vi "DriveModuleControl_TravTunePID-ALT.vi"(8 "error in":errorcluster, 9 "Actual State":T1={"Speed"=0.0, "Angle"={"VALUE"=0.0, "COS"=1.0, "SIN"=0.0}} {"Angle"."SIN" format="%13.4f"; "Angle"."COS" format="%13.4f"; "Angle"."VALUE" format="%13.4f"}, 10 "Desired State":T1={"Speed"=0.0, "Angle"={"VALUE"=0.0, "COS"=1.0, "SIN"=0.0}} {"Angle"."SIN" format="%13.4f"; "Angle"."COS" format="%13.4f"; "Angle"."VALUE" format="%13.4f"}, 11 "ModualNamePrefix":i32) -> (0 "error out":errorcluster)   [LabVIEW 2023]
uses:
  <vilib>/Rock Robotics/WPI/ThirdParty/JAS_Junk/TrajLib/TypeDef/SWERVE_DRIVE_MODULE_STATE.ctl
  <vilib>/Rock Robotics/WPI/ThirdParty/JAS_Junk/TrajLib/TypeDef/ROTATION2D.ctl
  <vilib>/Rock Robotics/WPI/ThirdParty/JAS_Junk/TrajLib/Rotation2d_Minus.vi
  <vilib>/Rock Robotics/WPI/ThirdParty/JAS_Junk/TrajLib/Rotation2d_GetRadians.vi
  <vilib>/Rock Robotics/WPI/ThirdParty/JAS_Junk/TrajLib/SwerveModuleState_New.vi
  <vilib>/Rock Robotics/WPI/ThirdParty/JAS_Junk/TrajLib/Rotation2d_RotateBy.vi
  <vilib>/Rock Robotics/WPI/ThirdParty/JAS_Junk/TrajLib/Rotation2d_CreateAngle.vi
  <vilib>/Rock Robotics/WPI/ThirdParty/JAS_Junk/TrajLib/SimpleMotorFF_Calculate.vi
  <vilib>/Rock Robotics/WPI/ThirdParty/JAS_Junk/TrajLib/PIDController_AtSetpoint.vi
  <vilib>/Rock Robotics/WPI/ThirdParty/JAS_Junk/TrajLib/PIDController_SetPIDF.vi
  <vilib>/Rock Robotics/WPI/ThirdParty/JAS_Junk/TrajLib/PIDController_SetDerivativeFilter.vi
  <vilib>/Rock Robotics/WPI/ThirdParty/JAS_Junk/TrajLib/PIDController_SetIntegratorRange.vi
  <vilib>/Rock Robotics/WPI/ThirdParty/JAS_Junk/TrajLib/PIDController_SetTolerancePandV.vi
  <vilib>/Rock Robotics/WPI/ThirdParty/JAS_Junk/TrajLib/PIDController_DisableContinousInput.vi
  <vilib>/Rock Robotics/WPI/ThirdParty/JAS_Junk/TrajLib/PIDController_EnableContinousInput.vi
  <vilib>/Rock Robotics/WPI/ThirdParty/JAS_Junk/TrajLib/PIDController_Reset.vi
  <vilib>/Rock Robotics/WPI/ThirdParty/JAS_Junk/TrajLib/PIDController_New.vi
  <vilib>/Rock Robotics/WPI/ThirdParty/JAS_Junk/TrajLib/PIDController_SetOutputLimits.vi
  <vilib>/Rock Robotics/WPI/ThirdParty/JAS_Junk/TrajLib/VI/PIDController_SetIntegratorZone.vi
  <vilib>/Rock Robotics/WPI/ThirdParty/JAS_Junk/TrajLib/Conv_Radians_Deg.vi
  <vilib>/Rock Robotics/WPI/ThirdParty/JAS_Junk/TrajLib/Rotation2d_UnaryMinus.vi
  <vilib>/Rock Robotics/WPI/ThirdParty/JAS_Junk/TrajLib/Rotation2d_CreateXY.vi
  <vilib>/Rock Robotics/WPI/ThirdParty/JAS_Junk/TrajLib/PIDController_NewPeriod.vi
  <vilib>/Rock Robotics/WPI/ThirdParty/JAS_Junk/TrajLib/Util_CalcDist.vi
  <vilib>/Rock Robotics/SystemInterfaces/NetworkCommunication/NetComm_UsageReport_report.vi
  DriveGlobal.vi
  <vilib>/Rock Robotics/WPI/ThirdParty/Phoenix6/Phoenix6_Device_RefNumRegistryGet.vi
  <vilib>/Rock Robotics/WPI/MotorControl/WPI_MotorControlRefNum Registry Get.vi
  <vilib>/Rock Robotics/Network Tables/NT Write Number.vi
  <vilib>/Rock Robotics/WPI/ThirdParty/JAS_Junk/TrajLib/Globals/Util_LibraryGlobals.vi
  <vilib>/Rock Robotics/WPI/ThirdParty/JAS_Junk/TrajLib/PIDController_AdvCalculate_FF_Sp_Pv.vi
  <vilib>/Rock Robotics/WPI/ThirdParty/JAS_Junk/TrajLib/Trajectory_Library.lvlib
  <vilib>/Rock Robotics/WPI/ThirdParty/REV Robotics/REVLib/Typedef/Spark MAX Control Type.ctl
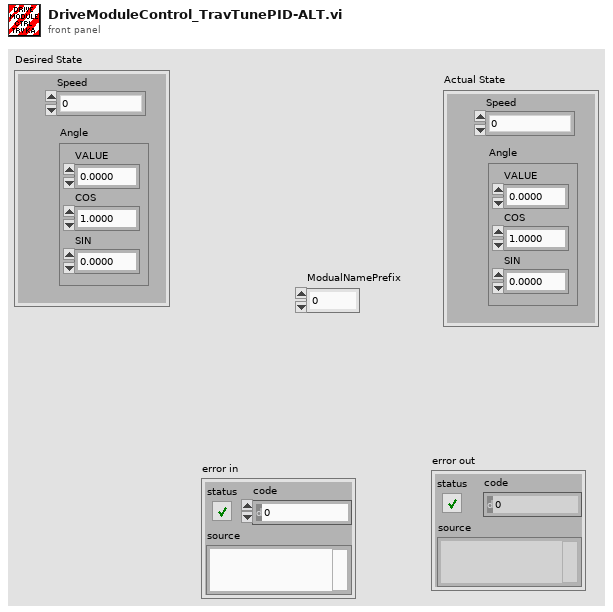
[diagram p1: front panel]
types:
  T1 = typedef "Trajectory_Library.lvlib/SWERVE_DRIVE_MODULE_STATE.ctl" = cluster{"Speed":dbl, "Angle":T2}
  T2 = typedef "Trajectory_Library.lvlib/ROTATION2D.ctl" = cluster{"VALUE":dbl, "COS":dbl, "SIN":dbl}
  T3 = typedef "Spark MAX Control Type.ctl" = enum16{"Percent VBus", "Voltage", "Velocity", "Position", "Smart Motion", "Current", "Smart Velocity", "MAXMotion Position", "MAXMotion Velocity"}
  T4 = enum16{"Ziegler Nicols - Fast", "Ziegler Nicols - Normal", "Ziegler Nicols - Slow", "CHR regulator - 0% overshoot", "CHR regulator - 20% overshoot", "CHR servo - 0 % overshoot", "CHR servo - 20% overshoot"}
  T5 = typedef "WPI_MotorControlDeviceRef.ctl" = cluster{"DeviceStatus":errorcluster, "Type":T6, "PWM":cluster{"PWM Channel":T7, "DeadBand":T8}, "CAN":cluster{"Device Number":u8, "SetOutput VI Ref":variant, "GetOutput VI Ref":variant, "Enable VI Ref":variant, "Disable VI Ref":variant, "Data":variant}, "Invert":bool, "DIO PWM":cluster{"PWM \"Enable\" Channel":T7, "DIOChannel":T9, "PWM Rate":dbl}}
  T6 = typedef "WPI_MotorControlType.ctl" = enum16{"PWM", "CAN", "DIO PWM"}
  T7 = typedef "FPGA_DIOPWMChannel.ctl" = enum8{"PWM 0", "PWM 1", "PWM 2", "PWM 3", "PWM 4", "PWM 5", "PWM 6", "PWM 7", "PWM 8", "PWM 9", "PWM MXP 0", "PWM MXP 1", "PWM MXP 2", "PWM MXP 3", "PWM MXP 4", "PWM MXP 5", "PWM MXP 6", "PWM MXP 7", "PWM MXP 8", "PWM MXP 9", "Invalid"}
  T8 = typedef "WPI_PWMDeadband.ctl" = cluster{"Name":string, "maxPositivePwm":i32, "minPositivePwm":i32, "centerPwm":i32, "maxNegativePwm":i32, "minNegativePwm":i32, "angularRange":u16}
  T9 = typedef "FPGA_DIOChannel.ctl" = enum8{"DIO 0", "DIO 1", "DIO 2", "DIO 3", "DIO 4", "DIO 5", "DIO 6", "DIO 7", "DIO 8", "DIO 9", "DIO MXP 0", "DIO MXP 1", "DIO MXP 2", "DIO MXP 3", "DIO MXP 4", "DIO MXP 5", "DIO MXP 6", "DIO MXP 7", "DIO MXP 8", "DIO MXP 9", "DIO MXP 10", "DIO MXP 11", "DIO MXP 12", "DIO MXP 13", "DIO MXP 14", "DIO MXP 15", "SPI Port CS1", "SPI Port CS2", "SPI Port CS3", "SPI Port MISO", "SPI Port MOSI", "Invalid"}
  T10 = typedef "Trajectory_Library.lvlib/SIMPLE_MOTOR_FF.ctl" = cluster{"Ks":dbl, "Kv":dbl, "Ka":dbl, "KnInv":dbl}
  T11 = typedef "Trajectory_Library.lvlib/PID_ADV_LIMITS.ctl" = cluster{"MaxInput":dbl, "MinInput":dbl, "Continuous":bool, "MaxOutput":dbl, "MinOutput":dbl}
  T12 = typedef "Trajectory_Library.lvlib/PID_ADV_TUNING.ctl" = cluster{"Kf":dbl, "Kp":dbl, "Ki":dbl, "Kd":dbl, "MaximumIntegral":dbl, "MinimumIntegral":dbl, "Filter Derivative":bool, "IntegralZone":dbl}
  T13 = cluster{"Controller Constant Type":enum16{"Ziegler Nicols - Fast", "Ziegler Nicols - Normal", "Ziegler Nicols - Slow", "CHR regulator - 0% overshoot", "CHR regulator - 20% overshoot", "CHR servo - 0 % overshoot", "CHR servo - 20% overshoot"}, "Type of Controller":enum16{"P", "PI", "PID"}, "CO Offset":dbl, "Kn":dbl, "Tuning Tolerance":dbl, "Plant Tolerance":dbl, "Newest Avg Time ":i32, "Long Ave Time":i32}
  T14 = cluster{"Plant Gain (K)":dbl, "Time Constant (T)":dbl, "Dead Time (L)":dbl, "stimulus operating point":dbl, "response operating point":dbl}
  T15 = cluster{"proportional gain (Kp)":dbl, "integral time (Ki / Sec)":dbl, "derivative time (Kd /Sec)":dbl}
  T16 = cluster{"Const Done":bool, "Plant Done":bool, "PV Std Dev":dbl, "CO Std Dev":dbl}
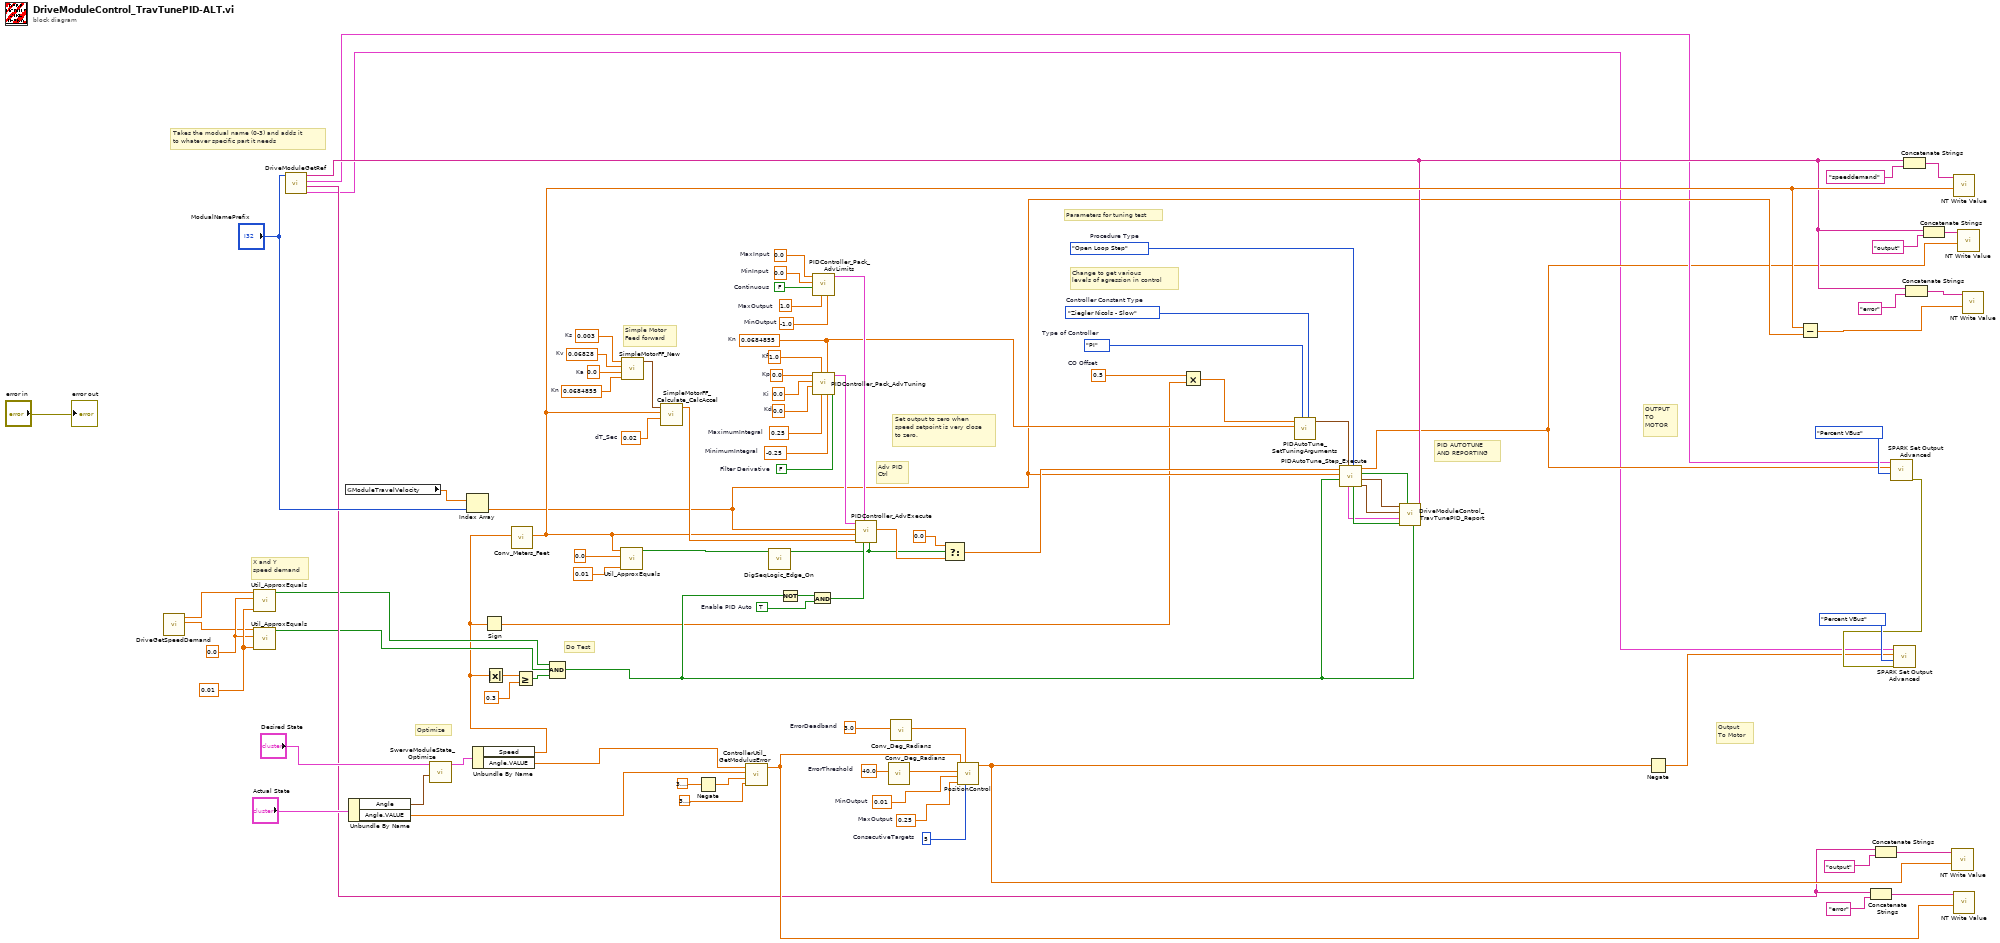
[diagram p0: block diagram]
diagram:
  w20 = 0.01 ("Tolerance")
  w19 = 0.0 ("Value 2")
  w32 = enum16{"Open Loop Step", "Closed Loop Step"}."Open Loop Step"  # Procedure Type
  w33 = T4."Ziegler Nicols - Slow"  # Controller Constant Type
  w34 = enum16{"P", "PI", "PID"}."PI"  # Type of Controller
  w14 = 0.5  # CO Offset
  w40 = TRUE  # Enable PID Auto
  w31 = 0.0684855  # Kn
  w66 = 0.0  # Kp
  w65 = 0.0  # Ki
  w64 = 0.0  # Kd
  w63 = 1.0  # Kf
  w62 = 0.25  # MaximumIntegral
  w61 = -0.25  # MinimumIntegral
  w60 = FALSE  # Filter Derivative
  w58 = 0.0  # MinInput
  w57 = FALSE  # Continuous
  w56 = 1.0  # MaxOutput
  w59 = -1.0  # MinOutput
  w55 = 0.0  # MaxInput
  w72 = 0.0684855  # Kn
  w71 = 0.02  # dT_Sec
  w69 = 0.003  # Ks
  w68 = 0.06828  # Kv
  w67 = 0.0  # Ka
  w81 = 5  # ConsecutiveTargets
  w78 = 0.25  # MaxOutput
  w82 = 0.01  # MinOutput
  w75 = 40.0  # ErrorThreshold
  w77 = 3.0  # ErrorDeadband
  # "X and Y \nspeed demand"
  # "Output\nTo Motor"
  # "OUTPUT\nTO \nMOTOR"
  # "PID AUTOTUNE\nAND REPORTING"
  # "Change to get various\nlevels of agression in control"
  # "Parameters for tuning test"
  # "Do Test"
  # "Optimize"
  # "Set output to zero when\nspeed setpoint is very close\nto zero."
  # "Adv PID\nCtrl"
  # "Simple Motor\nFeed forward"
  # "Takes the modual name (0-3) and adds it \nto whatever specific part it needs"
  n1 = call "DriveGetSpeedDemand.vi"() -> ("vY"=w17:dbl, "vX"=w18:dbl)  [unwired: 8 in, 2 out]
  n2 = call <vilib>:"Util_ApproxEquals.vi"("Tolerance"=w20, "Value 2"=w19, "Value 1"=w18) -> ("ApproxEquals"=w16:bool)  [unwired: 8 in]
  n3 = call <vilib>:"Util_ApproxEquals.vi"("Tolerance"=w20, "Value 2"=w19, "Value 1"=w17) -> ("ApproxEquals"=w15:bool)  [unwired: 8 in]
  n4 = call "DriveModuleGetRef.vi"("ModualNamePrefix"="ModualNamePrefix") -> ("SpinMot"=w2:T5, "SpinStr"=w46:string, "TravMot"=w4:T5, "TravStr"=w26:string)  [unwired: 5 in, 2 out]
  n5 = global read "DriveGlobal.vi" "ModuleTravelVelocity"() -> (w51:dbl[])
  n6 = Unbundle By Name("Actual State") -> ("Angle"=w88:T2, "Angle.VALUE"=w85:dbl)
  n7 = call <vilib>:"SwerveModuleState_Optimize.vi"("CurrentAngle"=w88, "Desired State"="Desired State") -> ("out SWERVE_DRIVE_MODULE_STATE"=w86:T1)  [unwired: 9 in]
  n8 = Index Array(array=w51, index="ModualNamePrefix") -> (element=w23:dbl)
  n9 = Unbundle By Name(w86) -> ("Speed"=w12:dbl, "Angle.VALUE"=w10:dbl)
  n10 = Sign(1:w12) -> (0:w11:dbl)
  n11 = Absolute Value(x=w12) -> (abs(x)=w37:dbl)
  n12 = call <vilib>:"Conv_Meters_Feet.vi"("Meters"=w12) -> ("Feet"=w43:dbl)  [unwired: 10 in]
  n13 = Greater Or Equal?(x=w37, y=0.3) -> (x >= y?=w22:bool)
  n14 = Compound Arithmetic op=AND(w16, w15, w22) -> (w21:bool)
  n15 = call <vilib>:"Util_ApproxEquals.vi"("Tolerance"=0.01, "Value 2"=0.0, "Value 1"=w43) -> ("ApproxEquals"=w9:bool)  [unwired: 8 in]
  n16 = call <vilib>:"SimpleMotorFF_New.vi"("Kn"=w72, "Ka"=w67, "Kv"=w68, "Ks"=w69) -> ("SIMPLE_MOTOR_FF"=w70:T10)  [unwired: 7 in]
  n17 = call <vilib>:"SimpleMotorFF_Calculate_CalcAccel.vi"("dT_Sec"=w71, "VelSp"=w43, "SIMPLE_MOTOR_FF"=w70) -> ("FeedForward"=w52:dbl)  [unwired: 8 in]
  n18 = Negate(x=3.141592653589793) -> (-x=w87:dbl)
  n19 = call <vilib>:"ControllerUtil_GetModulusError.vi"("Maximum_Input"=3.141592653589793, "Minimum_Input"=w87, "Measurerment(PV)"=w85, "Reference(SP)"=w10) -> ("Error"=w79:dbl)  [unwired: 7 in]
  n20 = call <vilib>:"DigSeqLogic_Edge_On.vi"("Input"=w9) -> ("On Edge"=w8:bool)  [unwired: 10 in]
  n21 = Not(x=w21) -> (.not. x?=w41:bool)
  n22 = And(x=w41, y=w40) -> (x .and. y?=w42:bool)
  n23 = call <vilib>:"PIDController_Pack_AdvLimits.vi"("MinOutput"=w59, "MaxOutput"=w56, "Continuous"=w57, "MinInput"=w58, "MaxInput"=w55) -> ("Adv PID Limits"=w53:T11)  [unwired: 6 in]
  n24 = call <vilib>:"PIDController_Pack_AdvTuning.vi"("Filter Derivative"=w60, "MinimumIntegral"=w61, "Kn"=w31, "MaximumIntegral"=w62, "Kf"=w63, "Kd"=w64, "Ki"=w65, "Kp"=w66) -> ("Adv PID Tuning"=w54:T12)  [unwired: 3 in]
  n25 = call <vilib>:"PIDController_AdvExecute.vi"("Reset"=w8, "Auto"=w42, "Adv PID Limits"=w53, "FF-FeedForward"=w52, "SP-SetPoint"=w43, "PV-Measurement"=w23, "Adv PID Tuning"=w54) -> ("CO-ControlOutput"=w39:dbl)  [unwired: 2 in, 2 out]
  n26 = call <vilib>:"Conv_Deg_Radians.vi"("Degress"=w75) -> ("Radians"=w74:dbl)  [unwired: 10 in]
  n27 = call <vilib>:"Conv_Deg_Radians.vi"("Degress"=w77) -> ("Radians"=w76:dbl)  [unwired: 10 in]
  n28 = Select(t=0.0, s=w8, f=w39) -> (s? t:f=w30:dbl)
  n29 = call "PositionControl.vi"("ConsecutiveTargets"=w81, "ErrorDeadband"=w76, "MaxOutput"=w78, "MinOutput"=w82, "ErrorThreshold"=w74, "Error"=w79) -> ("OutputValue"=w73:dbl)  [unwired: 3 in, 2 out]
  n30 = Multiply(x=w14, y=w11) -> (x*y=w13:dbl)
  n31 = call <vilib>:"PIDAutoTune_SetTuningArguments.vi"("Controller Constant Type"=w33, "Type of Controller"=w34, "Kn"=w31, "CO Offset"=w13) -> ("Configuration Parameters"=w35:T13)  [unwired: 7 in]
  n32 = call <vilib>:"PIDAutoTune_Step_Execute.vi"("Procedure Type"=w32, "Configuration Parameters"=w35, "Tune"=w21, "Measurement  (PV)"=w23, "Control Output (Co)"=w30) -> ("Plant and Test Data"=w28:T14, "New Tuning Parameters"=w29:T15, "Tuning Done"=w27:bool, "Adj CO"=w3:dbl, "Error Occured"=w25:bool, "Diagnostic Info"=w24:T16)  [unwired: 1 in]
  n33 = call "DriveModuleControl_TravTunePID_Report.vi"("Network Table Prefix"=w26, "TestInProgress"=w21, "Tuning Done"=w27, "Error Occured"=w25, "Diagnostic Info"=w24, "Plant and Test Data"=w28, "New Tuning Parameters"=w29) -> ()  [unwired: 5 in]
  n34 = Negate(x=w73) -> (-x=w1:dbl)
  n35 = Subtract(x=w43, y=w23) -> (x-y=w47:dbl)
  n36 = Concatenate Strings(w46, "error" ("refnum name")) -> (w92:string)
  n37 = Concatenate Strings(w46, "output" ("refnum name")) -> (w80:string)
  n38 = call <vilib>:"SPARK Set Output Advanced.vi"("Control Mode"=Spark_MAX_Control_Type."Percent VBus", "Setpoint"=w3, "MotorControlDevRef"=w4) -> ("error out"=w5:errorcluster)  [unwired: 7 in, 1 out]
  n39 = call <vilib>:"SPARK Set Output Advanced.vi"("error in (no error)"=w5, "Control Mode"=Spark_MAX_Control_Type."Percent VBus", "Setpoint"=w1, "MotorControlDevRef"=w2) -> ()  [unwired: 6 in, 2 out]
  n40 = Concatenate Strings(w26, "speeddemand" ("refnum name")) -> (w96:string)
  n41 = Concatenate Strings(w26, "error" ("refnum name")) -> (w48:string)
  n42 = Concatenate Strings(w26, "output" ("refnum name")) -> (w94:string)
  n43 = call-poly <vilib>:"NT Write Value.vi"("value"=w73, "name"=w80) -> ()  [unwired: 9 in, 1 out]
  n44 = call-poly <vilib>:"NT Write Value.vi"("value"=w43, "name"=w96) -> ()  [unwired: 9 in, 1 out]
  n45 = call-poly <vilib>:"NT Write Value.vi"("value"=w79, "name"=w92) -> ()  [unwired: 9 in, 1 out]
  n46 = call-poly <vilib>:"NT Write Value.vi"("value"=w3, "name"=w94) -> ()  [unwired: 9 in, 1 out]
  n47 = call-poly <vilib>:"NT Write Value.vi"("value"=w47, "name"=w48) -> ()  [unwired: 9 in, 1 out]
  "error out" <- "error in"
